vi "To Variant.vi"(0 "Obj in":refnum<class "Filter.lvclass">, 11 "error in (no error)":errorcluster) -> (4 "Obj out":refnum<class "Filter.lvclass">, 8 "Array":variant[](array[variant]), 15 "error out":errorcluster)   [LabVIEW 2020, in "Filter.lvclass"]
uses:
  Filter.lvclass
  Filter.lvclass/Filter.ctl
  Koop/KObject Class/KObject.lvclass
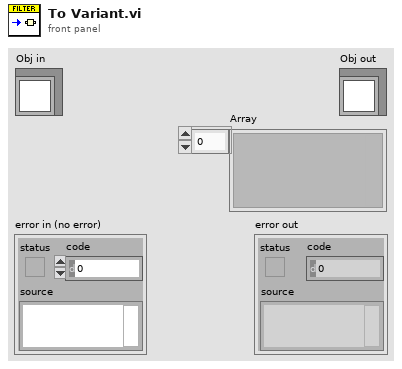
[diagram p1: front panel]
types:
  T1 = typedef "Filter.lvclass/Serialized.ctl" = cluster{"Type":T2, "CF (kHz)":dbl, "BW (kHz)":dbl, "Units":T3, "Class":T4, "Order":i32, "Cascade":bool}
  T2 = typedef "Filter.lvclass/Shape.ctl" = enum16{"OFF", "Lowpass", "Highpass", "Bandpass", "Bandstop"}
  T3 = typedef "Filter.lvclass/Units.ctl" = enum16{"Linear", "Octaves", "Min-Max"}
  T4 = typedef "Filter.lvclass/Class.ctl" = enum16{"Elliptic", "Butterworth", "Brickwall"}
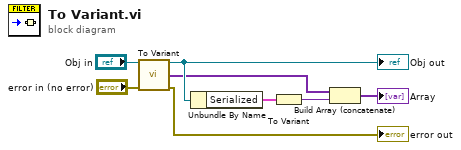
[diagram p0: block diagram]
diagram:
  n1 = call-parent "To Variant.vi"("KObject in"="Obj in", "error in (no error)"="error in (no error)") -> ("KObject out"=w3:refnum<class "Filter.lvclass">, "Array"=w2:variant[], "error out"=→"error out":errorcluster)  [unwired: 11 in]
  "Obj out" <- w3
  n2 = Unbundle By Name(w3) -> ("Serialized"=w4:T1)
  n3 = To Variant(anything=w4) -> (Variant=w5:variant)
  n4 = Build Array (concatenate)(w2, w5) -> (→"Array":variant[])
